vi "Next.vi"(8 "Error In":errorcluster, 11 "Reader In":refnum<class "Abstract.lvclass">) -> (0 "Error Out":errorcluster, 1 "Done":bool, 2 "Character":u8, 3 "Reader Out":refnum<class "Abstract.lvclass">)   [LabVIEW 2018, in "Toolkit.lvlib" / "Readers.lvlib" / "Abstract.lvclass"]
doc: "Reads the next character from a template."
uses:
  Abstract.lvclass
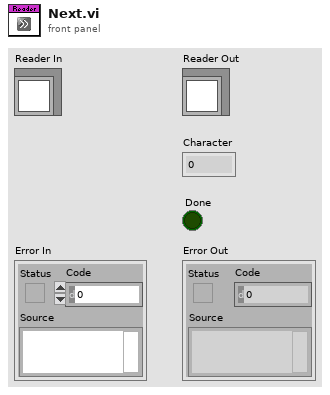
[diagram p1: front panel]
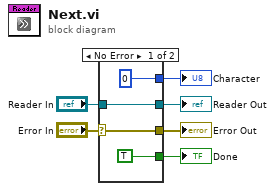
[diagram p0: block diagram]
diagram:
  n1 = case shown="No Error" "Error In" {
    selector: "Error In" -> [w9 w12]
    tunnel: [w9 w12] -> w5
    tunnel: [w10 w11] -> w3
    tunnel: "Reader In" -> [w10 w11]
    tunnel: [u8 0 _] -> w2
    tunnel: [TRUE ("Done") _] -> w1
    frame No Error {
    }
    frame Error {
    }
  }
  "Error Out" <- w5
  "Reader Out" <- w3
  "Character" <- w2
  "Done" <- w1
